vi "MasterVI.vi"() -> ()   [LabVIEW 2014]
uses:
  <vilib>/Analysis/NI_AALPro.lvlib
panel:
  out "SubVI Results":dbl[][](graph)
  out "A and B":dbl[][](graph)
  in  "Signal Specs":T1(array[cluster])=[{"signal type"=enum."sine", "frequency"=10.0, "amplitude"=3.0, "dc offset"=0.0, "phase"=10.0}, {"signal type"=enum."sine", "frequency"=5.0, "amplitude"=2.0, "dc offset"=0.0, "phase"=10.0}] {"phase" format="%0.2f"; "dc offset" format="%0.2f"; "amplitude" format="%0.2f"; "frequency" format="%0.2f"}
  in  "# of samples":i32=100
  # "A"
  # "B"
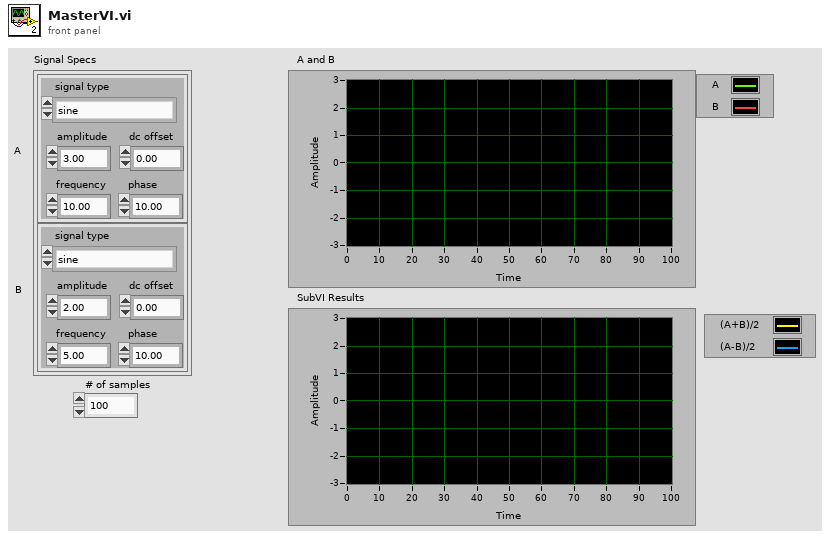
[diagram p1: front panel]
types:
  T1 = cluster{"signal type":enum16{"sine", "cosine", "triangle", "square", "sawtooth", "increasing ramp", "decreasing ramp"}, "frequency":dbl, "amplitude":dbl, "dc offset":dbl, "phase":dbl}[]
  T2 = enum16{"sine", "cosine", "triangle", "square", "sawtooth", "increasing ramp", "decreasing ramp"}
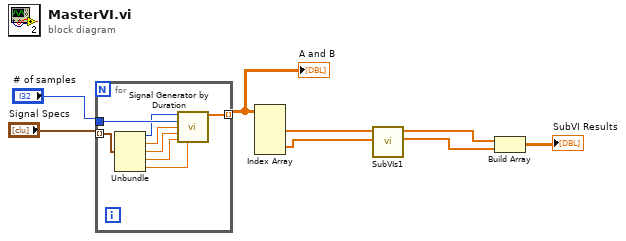
[diagram p0: block diagram]
diagram:
  n1 = for {
    tunnel: "# of samples" -> [w16]
    tunnel: "Signal Specs" -> [w15] mode=indexing
    tunnel: [w10] -> w6 mode=indexing
    n2 = Unbundle(w15) -> ("signal type"=w14:T2, "frequency"=w13:dbl, "amplitude"=w12:dbl, "dc offset"=w11:dbl, "phase"=w9:dbl)
    n3 = call <vilib>:"Signal Generator by Duration.vi"("signal type"=w14, "# of samples"=w16, "frequency"=w13, "amplitude"=w12, "dc offset"=w11, "phase in"=w9) -> ("signal"=w10:dbl[])  [unwired: 6 in, 3 out]
  }
  "A and B" <- w6
  n4 = Index Array(array=w6) -> (element #1=w5:dbl[], element #2=w4:dbl[])  [unwired: 4 in]
  n5 = call "SubVIs1.vi"("B"=w4, "A"=w5) -> ("(A-B)/2"=w3:dbl[], "(A+B)/2"=w2:dbl[])  [unwired: 8 in]
  n6 = Build Array(w2, w3) -> (→"SubVI Results":dbl[][])
